vi "Correction Collect Zero.vi"(8 "error in (no error)":errorcluster, 10 "Platform Slot Number (10)":i16=10 min=-1 max=255, 11 "VISA resource name":refnum<visa-resource-name>) -> (0 "error out":errorcluster, 3 "VISA resource name out":refnum<visa-resource-name>)   [LabVIEW 2018, in "LTB-1.lvlib" / "3150.lvlib"]
doc: "Performs the offset nulling on the internal power meter.\n\n<B>Note</B>\nThis command is applicable only for <B>Self-adjusting module</B> type of 3150. For standard module, \"Power control option not available.\" message will be returned as it doesn't support Output Power control mode. This command will take atleast 30 seconds to complete. Refer IQS-3150 user manual for more information."
uses:
  3150.lvlib
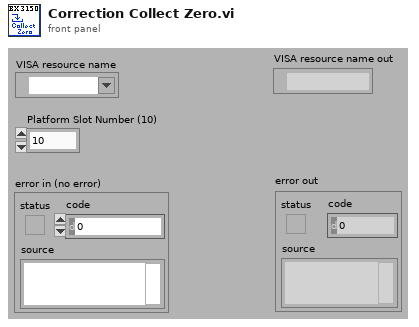
[diagram p1: front panel]
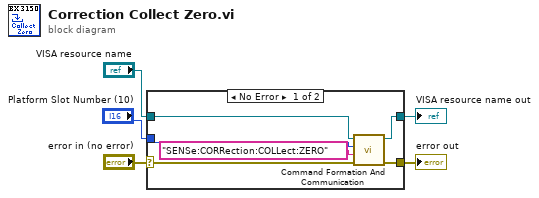
[diagram p0: block diagram]
diagram:
  n1 = case shown="No Error" "error in (no error)" {
    selector: "error in (no error)" -> [w10 w12]
    tunnel: "VISA resource name" -> [w11 w13]
    tunnel: [w9 w13] -> w3
    tunnel: [w8 w12] -> w2
    tunnel: "Platform Slot Number (10)" -> [w6 _]
    frame No Error {
      n2 = call "Command Formation And Communication.vi"("error in (no error)"=w10, "Command"="SENSe:CORRection:COLLect:ZERO", "Platform Slot Number"=w6, "VISA resource name"=w11) -> ("error out"=w8:errorcluster, "VISA resource name out"=w9:refnum<visa-resource-name>)  [unwired: 6 out]
    }
    frame Error {
    }
  }
  "VISA resource name out" <- w3
  "error out" <- w2
